vi "ZeroMQ_PUB.vi"() -> ()   [LabVIEW 2018]
uses:
  <vilib>/addons/zeromq/socket_type.ctl
  <vilib>/addons/zeromq/zeromq.lvlib
  <vilib>/addons/zeromq/zmq_socket.lvclass
  <vilib>/addons/zeromq/socket_options.ctl
  <vilib>/addons/zeromq/zmq_context.lvclass
panel:
  out "command":string
  in  "stop 3":bool
  out "error out 3":errorcluster
  out "pub":string
  out "error out 2":errorcluster
  out "sub":string
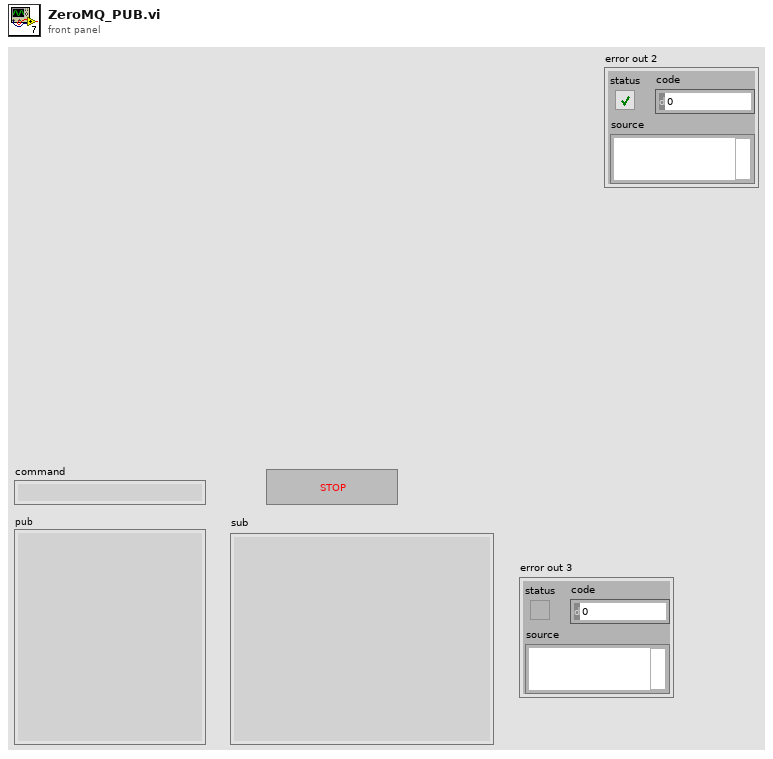
[diagram p1: front panel]
types:
  T1 = typedef "zeromq.lvlib/socket_type.ctl" = enum8{"ZMQ_PAIR", "ZMQ_PUB", "ZMQ_SUB", "ZMQ_REQ", "ZMQ_REP", "ZMQ_DEALER", "ZMQ_ROUTER", "ZMQ_PULL", "ZMQ_PUSH", "ZMQ_XPUB", "ZMQ_XSUB", "ZMQ_STREAM", "ZMQ_SERVER", "ZMQ_CLIENT", "ZMQ_RADIO", "ZMQ_DISH", "ZMQ_GATHER", "ZMQ_SCATTER", "ZMQ_DGRAM"}
  T2 = cluster{"ID":u32, "Address":string, "Service Name 1":string, "Service Name 2":string, "queue TX":refnum<queue>, "queue RX":refnum<queue>, "Port 1":u32, "Port 2":u32}
  T3 = typedef "zeromq.lvlib/socket_options.ctl" = enum8{"NONE", "ZMQ_HWM", "<2>", "ZMQ_SWAP", "ZMQ_AFFINITY", "ZMQ_ROUTING_ID", "ZMQ_SUBSCRIBE", "ZMQ_UNSUBSCRIBE", "ZMQ_RATE", "ZMQ_RECOVERY_IVL", "ZMQ_MCAST_LOOP", "ZMQ_SNDBUF", "ZMQ_RCVBUF", "ZMQ_RCVMORE", "ZMQ_FD", "ZMQ_EVENTS", "ZMQ_TYPE", "ZMQ_LINGER", "ZMQ_RECONNECT_IVL", "ZMQ_BACKLOG", "ZMQ_RECOVERY_IVL_MSEC", "ZMQ_RECONNECT_IVL_MAX", "ZMQ_MAXMSGSIZE", "ZMQ_SNDHWM", "ZMQ_RCVHWM", "ZMQ_MULTICAST_HOPS", "<26>", "ZMQ_RCVTIMEO", "ZMQ_SNDTIMEO", "<29>", "<30>", "ZMQ_IPV4ONLY", "ZMQ_LAST_ENDPOINT", "ZMQ_ROUTER_MANDATORY", "ZMQ_TCP_KEEPALIVE", "ZMQ_TCP_KEEPALIVE_CNT", "ZMQ_TCP_KEEPALIVE_IDLE", "ZMQ_TCP_KEEPALIVE_INTVL", "ZMQ_TCP_ACCEPT_FILTER", "ZMQ_IMMEDIATE", "ZMQ_XPUB_VERBOSE", "ZMQ_ROUTER_RAW", "ZMQ_IPV6", "ZMQ_MECHANISM", "ZMQ_PLAIN_SERVER", "ZMQ_PLAIN_USERNAME", "ZMQ_PLAIN_PASSWORD", "ZMQ_CURVE_SERVER", "ZMQ_CURVE_PUBLICKEY", "ZMQ_CURVE_SECRETKEY", "ZMQ_CURVE_SERVERKEY", "ZMQ_PROBE_ROUTER", "ZMQ_REQ_CORRELATE", "ZMQ_REQ_RELAXED", "ZMQ_CONFLATE", "ZMQ_ZAP_DOMAIN", "ZMQ_ROUTER_HANDOVER", "ZMQ_TOS", "ZMQ_IPC_FILTER_PID", "ZMQ_IPC_FILTER_UID", "ZMQ_IPC_FILTER_GID", "ZMQ_CONNECT_ROUTING_ID", "ZMQ_GSSAPI_SERVER", "ZMQ_GSSAPI_PRINCIPAL", "ZMQ_GSSAPI_SERVICE_PRINCIPAL", "ZMQ_GSSAPI_PLAINTEXT", "ZMQ_HANDSHAKE_IVL", "<67>", "ZMQ_SOCKS_PROXY", "ZMQ_XPUB_NODROP", "ZMQ_BLOCKY", "ZMQ_XPUB_MANUAL", "ZMQ_XPUB_WELCOME_MSG", "ZMQ_STREAM_NOTIFY", "ZMQ_INVERT_MATCHING", "ZMQ_HEARTBEAT_IVL", "ZMQ_HEARTBEAT_TTL", "ZMQ_HEARTBEAT_TIMEOUT", "ZMQ_XPUB_VERBOSER", "ZMQ_CONNECT_TIMEOUT", "ZMQ_TCP_MAXRT", "ZMQ_THREAD_SAFE", "<82>", "<83>", "ZMQ_MULTICAST_MAXTPDU", "ZMQ_VMCI_BUFFER_SIZE", "ZMQ_VMCI_BUFFER_MIN_SIZE", "ZMQ_VMCI_BUFFER_MAX_SIZE", "ZMQ_VMCI_CONNECT_TIMEOUT", "ZMQ_USE_FD", "ZMQ_GSSAPI_PRINCIPAL_NAMETYPE", "ZMQ_GSSAPI_SERVICE_PRINCIPAL_NAMETYPE", "ZMQ_BINDTODEVICE", "ZMQ_ZAP_ENFORCE_DOMAIN", "ZMQ_LOOPBACK_FASTPATH", "ZMQ_METADATA", "ZMQ_MULTICAST_LOOP", "ZMQ_ROUTER_NOTIFY"}
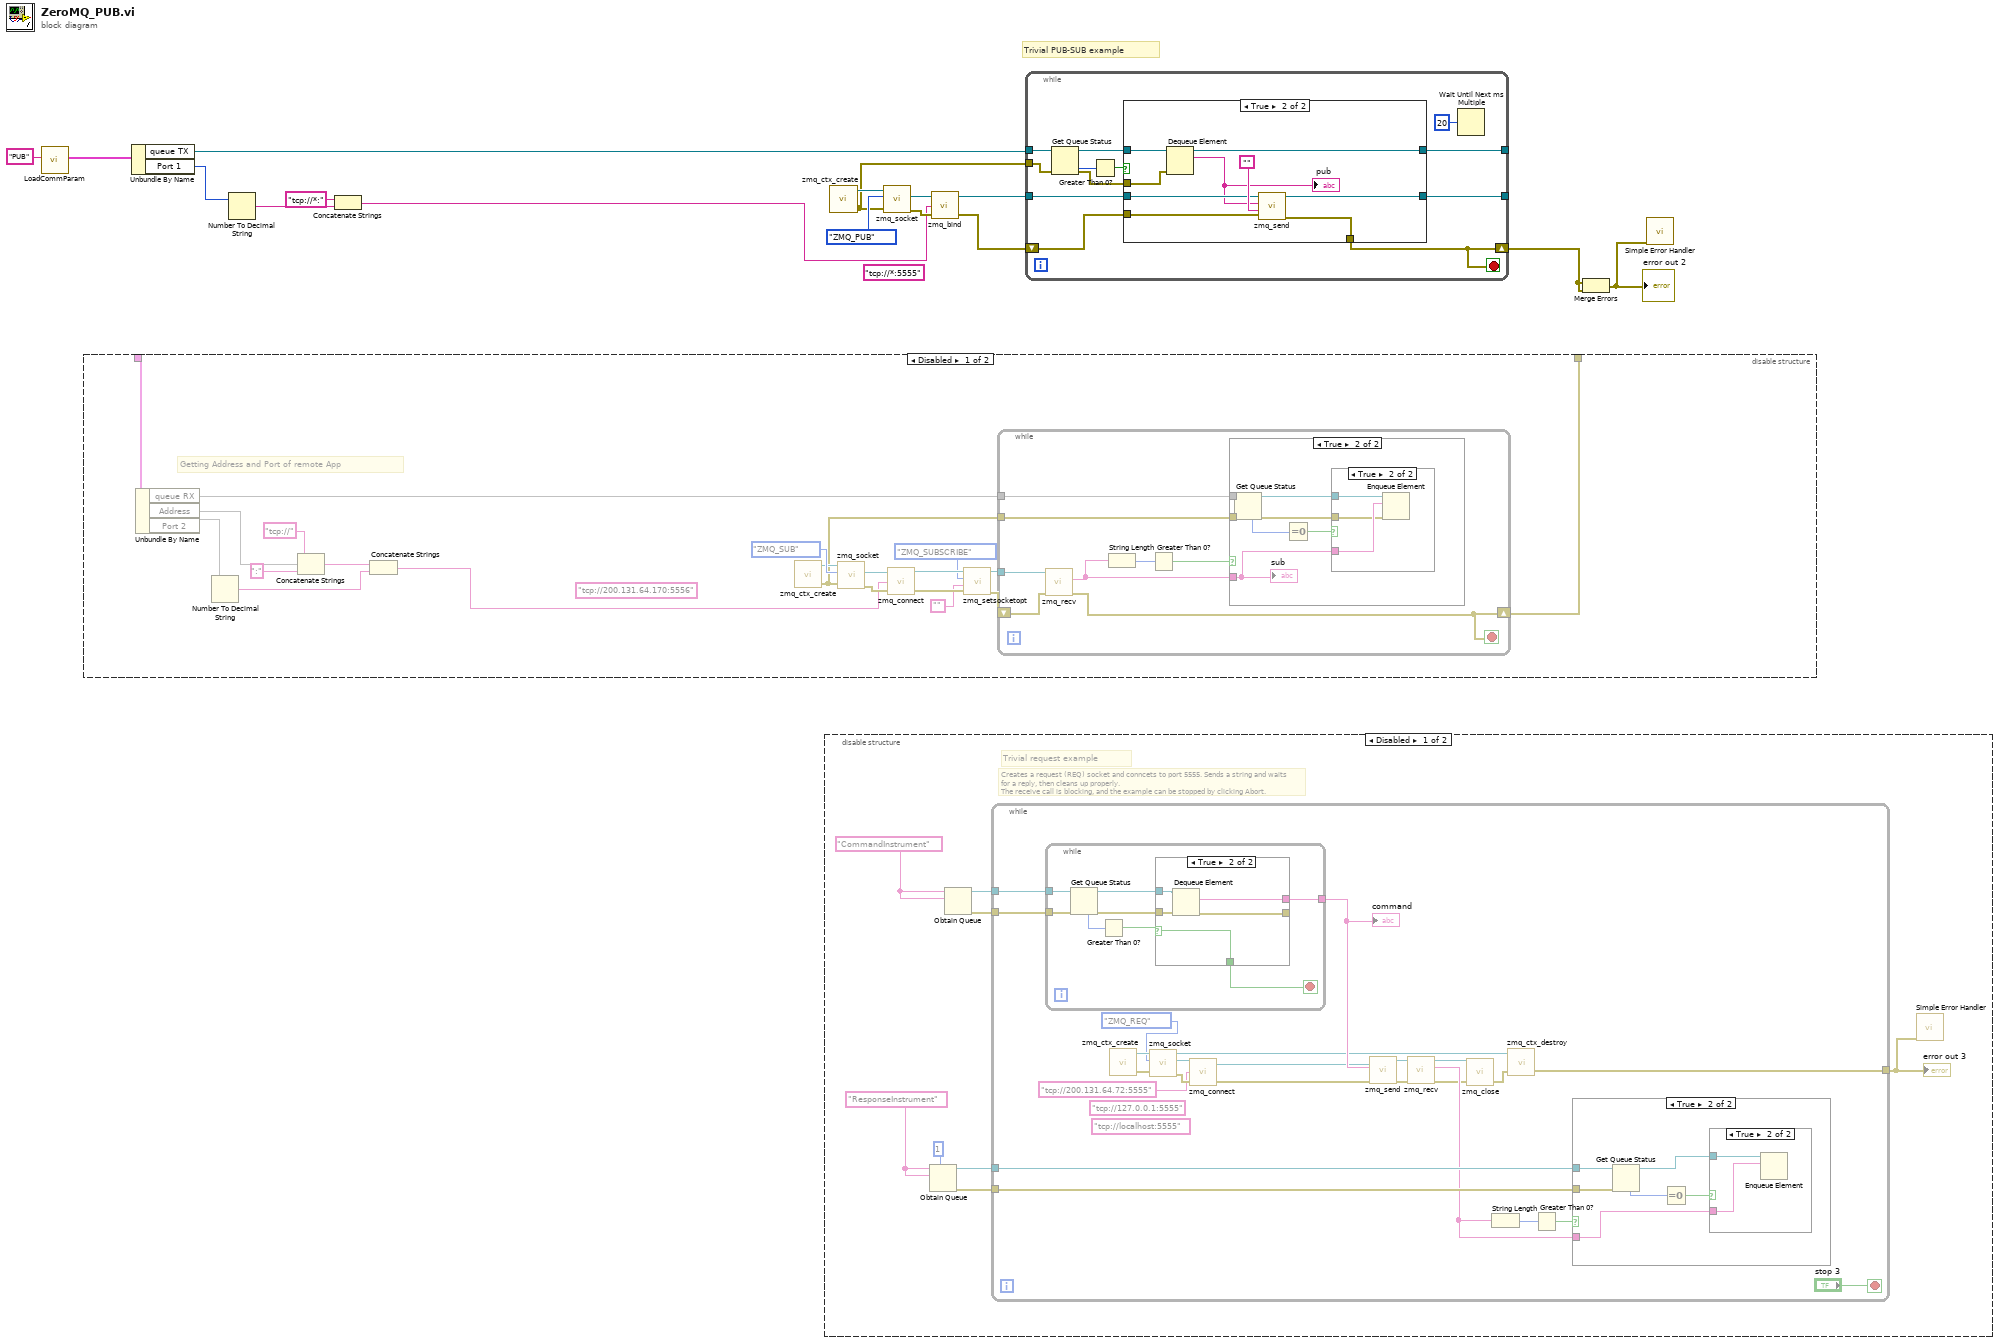
[diagram p0: block diagram]
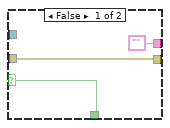
[diagram p8: hidden frame]
diagram:
  (unwired) "tcp://*:5555" ("endpoint")
  # "Trivial PUB-SUB example"
  n1 = call "LoadCommParam.vi"("section name"="PUB") -> ("output cluster"=w4:T2)  [unwired: 10 in]
  n2 = disable-structure shown="Disabled" {
    disable-tunnel: _ -> [w26 _]
    disable-tunnel: [w17 _] -> _
    frame Disabled {
      (unwired) "tcp://200.131.64.170:5556" ("endpoint")
      # "Getting Address and Port of remote App"
      n3 = Unbundle By Name(w26) -> ("queue RX"=w24, "Address"=w23, "Port 2"=w22)
      n4 = Number To Decimal String(number=w22) -> (decimal integer string=w21:string)  [unwired: 1 in]
      n5 = Concatenate Strings("tcp://" ("string"), w23, ":" ("string")) -> (w20:string)
      n6 = Concatenate Strings(w20, w21) -> (w27:string)
      n7 = call <vilib>:"zmq_ctx_create.vi"() -> ("error out"=w25:errorcluster, "context out"=w28:refnum<class "zmq_context.lvclass">)  [unwired: 4 in]
      n8 = call <vilib>:"zmq_socket.vi"("error in"=w25, "socket type"=socket_type."ZMQ_SUB", "context in"=w28) -> ("error out"=w36:errorcluster, "socket out"=w29:refnum<class "zmq_socket.lvclass">)  [unwired: 2 in, 1 out]
      n9 = call <vilib>:"zmq_connect.vi"("error in"=w36, "endpoint"=w27, "socket in"=w29) -> ("error out"=w34:errorcluster, "socket out"=w35:refnum<class "zmq_socket.lvclass">)  [unwired: 1 in]
      n10 = call <vilib>:"zmq_setsocketopt.vi"("error in"=w34, "value"="", "option"=socket_options."ZMQ_SUBSCRIBE", "socket in"=w35) -> ("error out"=w33:errorcluster, "socket out"=w32:refnum<class "zmq_socket.lvclass">)  [unwired: 2 in]
      n11 = while {
        tunnel: w32 -> [w38]
        tunnel: w24 -> [w41]
        shift-right: [w44] -> w17
        shift-left: w33 -> [w45]
        tunnel: w25 -> [w39]
        stop <- w44 stop-if-true
        n12 = call <vilib>:"zmq_recv.vi"("error in"=w45, "socket in"=w38) -> ("error out"=w44:errorcluster, "data"=w40:string)  [unwired: 3 in, 3 out]
        n13 = String Length(string=w40) -> (length=w43:i32)
        n14 = Greater Than 0?(x=w43) -> (x > 0?=w42:bool)
        n15 = case shown="True" w42 {
          tunnel: w41 -> [_ w51]
          tunnel: w40 -> [_ w48]
          tunnel: w39 -> [_ w47]
          frame False {
          }
          frame True {
            n16 = Get Queue Status(queue=w51, error in (no error)=w47) -> (queue out=w49:refnum<queue>, error out=w46:errorcluster, # elements in queue=w52:i32)  [unwired: 1 in, 5 out]
            n17 = Equal To 0?(x=w52) -> (x = 0?=w50:bool)
            n18 = case shown="True" w50 {
              tunnel: w49 -> [_ w55]
              tunnel: w48 -> [_ w54]
              tunnel: w46 -> [_ w53]
              frame False {
              }
              frame True {
                n19 = Enqueue Element(queue=w55, element=w54, error in (no error)=w53) -> ()  [unwired: 1 in, 3 out]
              }
            }
            "sub" <- w48
          }
        }
      }
    }
    frame Enabled {
    }
  }
  n20 = Unbundle By Name(w4) -> ("queue TX"=w5:refnum<queue>, "Port 1"=w9:u32)
  n21 = Number To Decimal String(number=w9) -> (decimal integer string=w8:string)  [unwired: 1 in]
  n22 = Concatenate Strings("tcp://*:" ("string"), w8) -> (w3:string)
  n23 = disable-structure shown="Disabled" {
    frame Disabled {
      w56 = "ResponseInstrument"
      w57 = "CommandInstrument"
      # "Creates a request (REQ) socket and conncets to port 5555. Sends a string and waits for a reply, then cleans up properly.\nThe receive call is blocking, and the example can be stopped by clicking Abort."
      # "Trivial request example"
      n24 = Obtain Queue(max queue size (-1, unlimited)=1, name (unnamed)=w56, element data type=w56) -> (queue out=w60:refnum<queue>, error out=w59:errorcluster)  [unwired: 2 in, 1 out]
      n25 = Obtain Queue(name (unnamed)=w57, element data type=w57) -> (queue out=w62:refnum<queue>, error out=w61:errorcluster)  [unwired: 3 in, 1 out]
      n26 = while {
        tunnel: w62 -> [w85]
        tunnel: w61 -> [w84]
        tunnel: w60 -> [w82]
        tunnel: w59 -> [w81]
        tunnel: [w68] -> w58
        stop <- "stop 3" stop-if-true
        (unwired) "tcp://127.0.0.1:5555" ("endpoint")
        (unwired) "tcp://localhost:5555" ("endpoint")
        n27 = while {
          tunnel: w85 -> [w102]
          tunnel: w84 -> [w101]
          tunnel: [w97] -> w83
          stop <- w96 stop-if-true
          n28 = Get Queue Status(queue=w102, error in (no error)=w101) -> (queue out=w98:refnum<queue>, error out=w99:errorcluster, # elements in queue=w103:i32)  [unwired: 1 in, 5 out]
          n29 = Greater Than 0?(x=w103) -> (x > 0?=w100:bool)
          n30 = case shown="True" w100 {
            selector: w100 -> [w104 w107]
            tunnel: w99 -> [w106 w111]
            tunnel: w98 -> [_ w110]
            tunnel: [w106 w109] -> _
            tunnel: ["" w108] -> w97
            tunnel: [w104 w107] -> w96
            frame False {
            }
            frame True {
              n31 = Dequeue Element(queue=w110, error in (no error)=w111) -> (element=w108:string, error out=w109:errorcluster)  [unwired: 1 in, 2 out]
            }
          }
        }
        "command" <- w83
        n32 = call <vilib>:"zmq_ctx_create.vi"() -> ("error out"=w73:errorcluster, "context out"=w76:refnum<class "zmq_context.lvclass">)  [unwired: 4 in]
        n33 = call <vilib>:"zmq_socket.vi"("error in"=w73, "socket type"=socket_type."ZMQ_REQ", "context in"=w76) -> ("error out"=w75:errorcluster, "socket out"=w74:refnum<class "zmq_socket.lvclass">, "context out"=w65:refnum<class "zmq_context.lvclass">)  [unwired: 2 in]
        n34 = call <vilib>:"zmq_connect.vi"("error in"=w75, "endpoint"="tcp://200.131.64.72:5555", "socket in"=w74) -> ("error out"=w70:errorcluster, "socket out"=w71:refnum<class "zmq_socket.lvclass">)  [unwired: 1 in]
        n35 = call <vilib>:"zmq_send.vi"("error in"=w70, "data"=w83, "socket in"=w71) -> ("error out"=w86:errorcluster, "socket out"=w87:refnum<class "zmq_socket.lvclass">)  [unwired: 4 in]
        n36 = call <vilib>:"zmq_recv.vi"("error in"=w86, "socket in"=w87) -> ("error out"=w67:errorcluster, "data"=w79:string, "socket out"=w66:refnum<class "zmq_socket.lvclass">)  [unwired: 3 in, 2 out]
        n37 = call <vilib>:"zmq_close.vi"("error in"=w67, "socket"=w66) -> ("error out"=w69:errorcluster)  [unwired: 3 in]
        n38 = String Length(string=w79) -> (length=w80:i32)
        n39 = call <vilib>:"zmq_ctx_destroy.vi"("error in"=w69, "context in"=w65) -> ("error out"=w68:errorcluster)  [unwired: 3 in]
        n40 = Greater Than 0?(x=w80) -> (x > 0?=w78:bool)
        n41 = case shown="True" w78 {
          tunnel: w82 -> [_ w92]
          tunnel: w79 -> [_ w89]
          tunnel: w81 -> [_ w88]
          frame False {
          }
          frame True {
            n42 = Get Queue Status(queue=w92, error in (no error)=w88) -> (queue out=w90:refnum<queue>, # elements in queue=w93:i32)  [unwired: 1 in, 6 out]
            n43 = Equal To 0?(x=w93) -> (x = 0?=w91:bool)
            n44 = case shown="True" w91 {
              tunnel: w90 -> [_ w95]
              tunnel: w89 -> [_ w94]
              frame False {
              }
              frame True {
                n45 = Enqueue Element(queue=w95, element=w94) -> ()  [unwired: 2 in, 3 out]
              }
            }
          }
        }
      }
      "error out 3" <- w58
      n46 = call <vilib>:"Simple Error Handler.vi"("error in (no error)"=w58) -> ()  [unwired: 4 in, 5 out]
    }
    frame Enabled {
    }
  }
  n47 = call <vilib>:"zmq_ctx_create.vi"() -> ("error out"=w6:errorcluster, "context out"=w16:refnum<class "zmq_context.lvclass">)  [unwired: 4 in]
  n48 = call <vilib>:"zmq_socket.vi"("error in"=w6, "socket type"=socket_type."ZMQ_PUB", "context in"=w16) -> ("error out"=w13:errorcluster, "socket out"=w14:refnum<class "zmq_socket.lvclass">)  [unwired: 2 in, 1 out]
  n49 = call <vilib>:"zmq_bind.vi"("error in"=w13, "endpoint"=w3, "socket in"=w14) -> ("error out"=w11:errorcluster, "socket out"=w12:refnum<class "zmq_socket.lvclass">)  [unwired: 1 in]
  n50 = while {
    tunnel: w12 -> [w119]
    tunnel: w5 -> [w123]
    tunnel: [w117] -> _
    tunnel: [w118] -> _
    tunnel: w6 -> [w116]
    shift-right: [w113] -> w1
    shift-left: w11 -> [w114]
    stop <- w113 stop-if-true
    n51 = Get Queue Status(queue=w123, error in (no error)=w116) -> (queue out=w122:refnum<queue>, error out=w115:errorcluster, # elements in queue=w121:i32)  [unwired: 1 in, 5 out]
    n52 = Greater Than 0?(x=w121) -> (x > 0?=w120:bool)
    n53 = case shown="True" w120 {
      tunnel: w122 -> [w125 w135]
      tunnel: w119 -> [w126 w133]
      tunnel: [w126 w131] -> w118
      tunnel: [w125 w132] -> w117
      tunnel: w115 -> [w124 w130]
      tunnel: [w124 w128] -> w113
      tunnel: w114 -> [_ w129]
      frame False {
      }
      frame True {
        n54 = Dequeue Element(queue=w135, error in (no error)=w130) -> (queue out=w132:refnum<queue>, element=w127:string)  [unwired: 1 in, 2 out]
        "pub" <- w127
        n55 = call <vilib>:"zmq_send.vi"("error in"=w129, "group"="", "data"=w127, "socket in"=w133) -> ("error out"=w128:errorcluster, "socket out"=w131:refnum<class "zmq_socket.lvclass">)  [unwired: 3 in]
      }
    }
    n56 = Wait Until Next ms Multiple(millisecond multiple=u32 20) -> ()  [unwired: 1 out]
  }
  n57 = Merge Errors(w1, w1) -> (w2:errorcluster)
  "error out 2" <- w2
  n58 = call <vilib>:"Simple Error Handler.vi"("error in (no error)"=w2) -> ()  [unwired: 4 in, 5 out]
